vi "Display.vi"(8 "error in":errorcluster, 11 "Input (DBL) in":refnum<class "Input (DBL).lvclass">) -> (0 "error out":errorcluster, 3 "Input (DBL) out":refnum<class "Input (DBL).lvclass">)   [LabVIEW 2021, in "Pop-Up.lvlib" / "Input (DBL).lvclass"]
doc: "This vi will display the input pop up waiting for a type Double input from the user\n\n<b>Code Developed By:</b>\nDaniel Coons\nTechnology Service Corporation\n1983 S Liberty Drive\nBloomington, IN 47403\nPhone: 812 558-7100\ndaniel.coons@tsc.com\nwww.tsc.com/atcs"
uses:
  Input (DBL).lvclass
  C:/Development/Open Source/tsc-pop-up/Popup/Popup.lvclass
  Input (DBL).lvclass/Input (DBL).ctl
  Popup/Popup.lvclass/Popup.ctl
  Popup/Data Member Access/Read Theme.vi
  Theme/Theme.lvclass
  Popup/Popup.lvclass
  user32.dll
panel:
  out "header":bool
  out "2D Picture":picture
  in  "OK Button":bool
  out "Input value out":dbl=1.0 min=1.0 format="%.10g"
  in  "Input":dbl format="%#.10g"
  out "String":string
  # "This VI displays the popup"
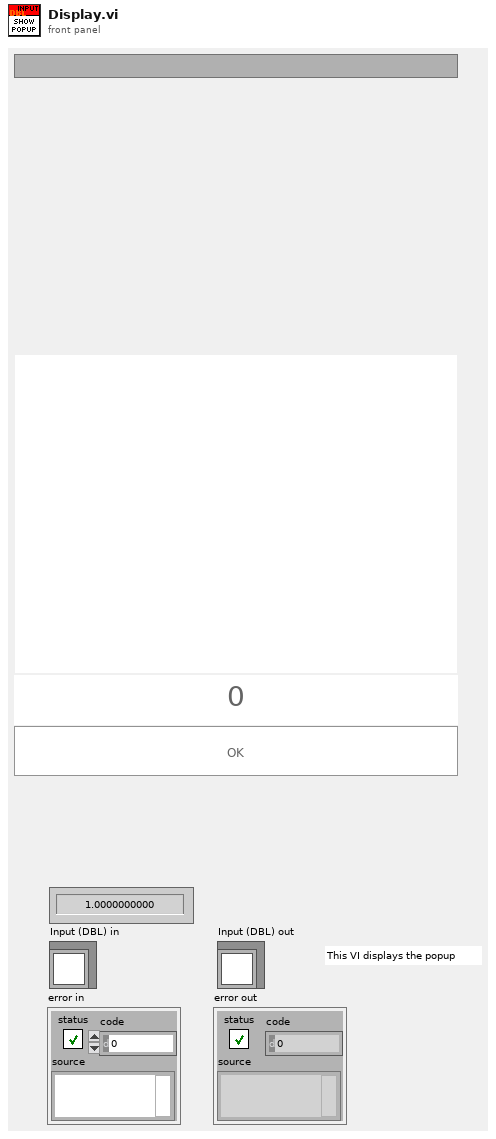
[diagram p1: front panel]
types:
  T1 = typedef "LVPoint32TypeDef.ctl" = cluster{"Horizontal":i32, "Vertical":i32}
  T2 = typedef "LVPositionTypeDef.ctl" = cluster{"Left":i32, "Top":i32}
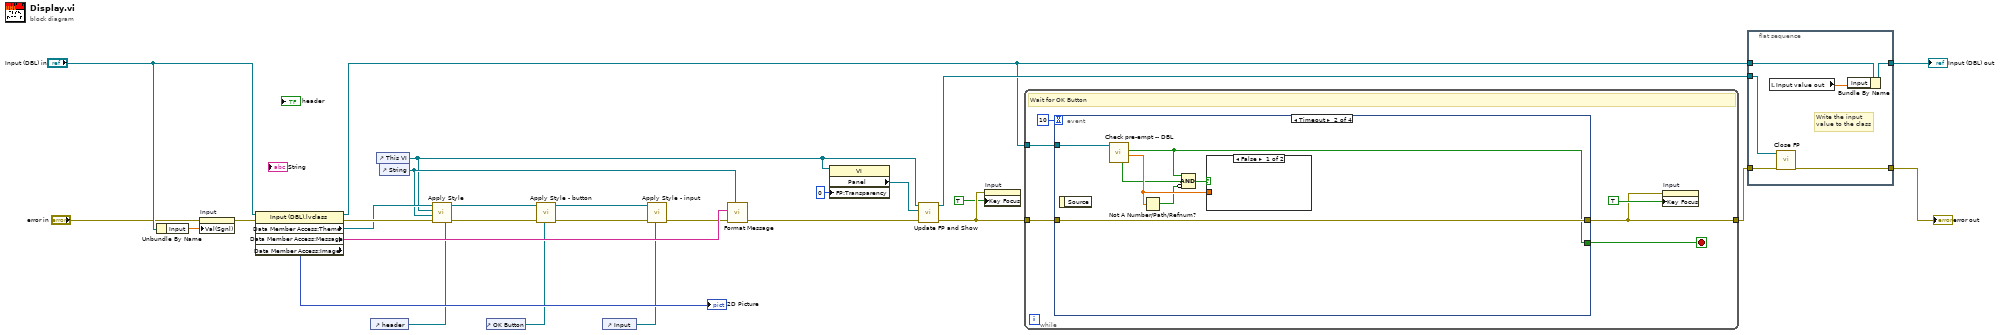
[diagram p0: block diagram]
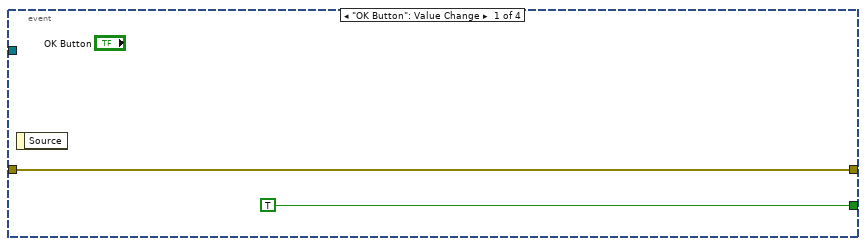
[diagram p2: hidden frame]
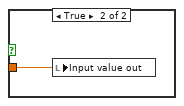
[diagram p3: hidden frame]
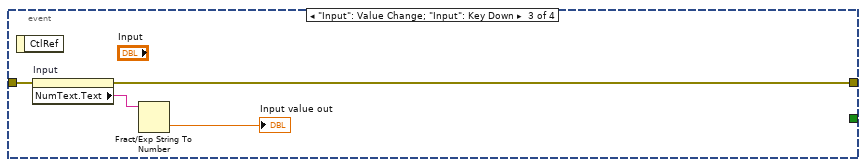
[diagram p4: hidden frame]
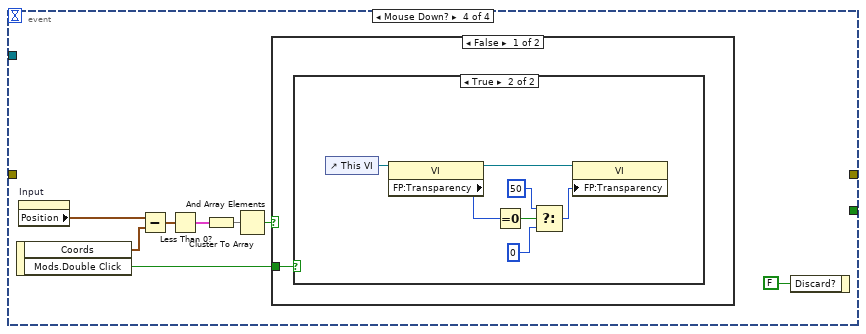
[diagram p5: hidden frame]
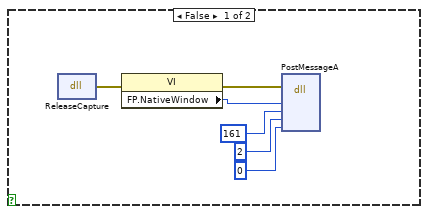
[diagram p6: hidden frame]
diagram:
  n1 = Unbundle By Name("Input (DBL) in") -> ("Input"=w22:dbl)
  n2 = property on="Input" class="DigNum (strict)"(error in="error in", "Val(Sgnl)"=w22) -> (error out=w23:errorcluster)  [unwired: 1 in, 1 out]
  n3 = property class="Input (DBL).lvclass"(reference="Input (DBL) in", error in=w23) -> (reference out=w17:refnum<class "Input (DBL).lvclass">, error out=w14:errorcluster, "Data Member Access:Theme"=w11:refnum<class "Theme.lvclass">, "Data Member Access:Message"=w15:string, "Data Member Access:Image"=→"2D Picture":picture)
  n4 = control-ref of="header"() -> (w8:refnum<vi>)
  n5 = control-ref of="This VI"() -> (w9:refnum<vi>)
  n6 = control-ref of="String"() -> (w10:refnum<vi>)
  n7 = call "Apply Style.vi"("header ref"=w8, "error in"=w14, "message ref"=w10, "pop up ref"=w9, "Theme in"=w11) -> ("error out"=w12:errorcluster, "Theme out"=w6:refnum<class "Theme.lvclass">)  [unwired: 5 in]
  n8 = control-ref of="OK Button"() -> (w5:refnum<vi>)
  n9 = call "Apply Style - button.vi"("button ref"=w5, "error in"=w12, "Theme in"=w6) -> ("error out"=w7:errorcluster, "Theme out"=w3:refnum<class "Theme.lvclass">)  [unwired: 7 in]
  n10 = control-ref of="Input"() -> (w2:refnum<vi>)
  n11 = call "Apply Style - input.vi"("input ref"=w2, "error in (no error)"=w7, "Theme in"=w3) -> ("error out"=w4:errorcluster)  [unwired: 7 in, 1 out]
  n12 = call "Format Message.vi"("formatted string"=w10, "error in"=w4, "String Input"=w15) -> ("error out"=w16:errorcluster)  [unwired: 7 in, 1 out]
  n13 = property class="VI"(reference=w9, "FP:Transparency"=u8 0 ("Front Panel Window:Transparency")) -> ("Panel"=w21:refnum<vi>)  [unwired: 1 in, 2 out]
  n14 = call "Update FP and Show.vi"("error in (no error)"=w16, "Panel Ref"=w21, "VI in"=w9) -> ("error out"=w19:errorcluster, "VI out"=w20:refnum<vi>)  [unwired: 7 in]
  n15 = property on="Input" class="DigNum (strict)"(error in=w19, "Key Focus"=TRUE) -> ()  [unwired: 1 in, 2 out]
  n16 = while {
    tunnel: w19 -> [w34]
    tunnel: [w29] -> w24
    tunnel: w17 -> [w31]
    stop <- w33 stop-if-true
    # "Wait for OK Button"
    n17 = event shown="[1] Timeout" {
      selector: _ -> [_ _ _ _]
      dyn-events: _ -> [_ _ _ _]
      timeout: 10 -> [_ _ _ _]
      tunnel: w34 -> [w36 w43 w48 _]
      tunnel: [w36 w43 w45 _] -> w29
      tunnel: [TRUE w40 _ _] -> w33
      tunnel: w31 -> [_ w42 _ _]
      event "OK Button": Value Change {
        n18 = event-data() -> ()  [unwired: 1 in, 1 out]
      }
      event Timeout {
        n19 = event-data() -> ()  [unwired: 1 in, 1 out]
        n20 = call "Check pre-empt -- DBL.vi"("_Popup in"=w42) -> ("Value?"=w41:dbl, "Pre-empted?"=w40:bool, "Type Match?"=w38:bool)  [unwired: 7 in, 1 out]
        n21 = Not A Number/Path/Refnum?(number/path/refnum=w41) -> (NaN/Path/Refnum?=w37:bool)
        n22 = Compound Arithmetic op=AND(w40, w38, invert w37) -> (w39:bool)
        n23 = case shown="False" w39 {
          tunnel: w41 -> [_ w44]
          frame False {
          }
          frame True {
            n24 = local write "Input value out"(w44) -> ()
          }
        }
      }
      event "Input": Value Change; "Input": Key Down {
        n25 = event-data() -> ()  [unwired: 1 in, 1 out]
        n26 = property on="Input" class="DigNum (strict)"(error in=w48) -> (error out=w45:errorcluster, "NumText.Text"=w47:string)  [unwired: 1 in, 1 out]
        n27 = Fract/Exp String To Number(string=w47) -> (number=→"Input value out":dbl)  [unwired: 3 in, 1 out]
      }
      event Mouse Down? {
        n28 = event-data() -> ("Coords"=w51:T1, "Mods.Double Click"=w49:bool)  [unwired: 1 in]
        n29 = property on="Input" class="DigNum (strict)"() -> ("Position"=w52:T2)  [unwired: 2 in, 2 out]
        n30 = Subtract(x=w52, y=w51) -> (x-y=w53:T2)
        n31 = Less Than 0?(x=w53) -> (x < 0?=w54:cluster{"Left":bool, "Top":bool})
        n32 = Cluster To Array(cluster=w54) -> (array=w55:bool[])
        n33 = And Array Elements(Boolean array=w55) -> (logical AND=w50:bool)
        n34 = case shown="False" w50 {
          tunnel: w49 -> [w57 _]
          frame False {
            n35 = case shown="True" w57 {
              frame False {
                n36 = dll-call lib="user32.dll" fn="ReleaseCapture"() -> (error out=w61:errorcluster)  [unwired: 4 in, 1 out]
                n37 = property class="VI"(error in=w61) -> (error out=w62:errorcluster, "FP.NativeWindow"=w63:u64)  [unwired: 1 in, 1 out]
                n38 = dll-call lib="user32.dll" fn="PostMessageA"(error in=w62, "hWnd"=w63, "Msg"=161, "wParam"=2, "lParam"=0) -> ()  [unwired: 7 in, 2 out]
              }
              frame True {
                n39 = control-ref of="This VI"() -> (w70:refnum<vi>)
                n40 = property class="VI"(reference=w70) -> (reference out=w68:refnum<vi>, "FP:Transparency"=w69:u8)  [unwired: 1 in, 1 out]
                n41 = Equal To 0?(x=w69) -> (x = 0?=w67:bool)
                n42 = Select(t=u8 50, s=w67, f=u8 0) -> (s? t:f=w66:u8)
                n43 = property class="VI"(reference=w68, "FP:Transparency"=w66) -> ()  [unwired: 1 in, 2 out]
              }
            }
          }
          frame True {
          }
        }
        n44 = event-data("Discard?"=FALSE) -> ()  [unwired: 1 in, 1 out]
      }
    }
    n45 = property on="Input" class="DigNum (strict)"(error in=w29, "Key Focus"=TRUE) -> ()  [unwired: 1 in, 2 out]
  }
  n46 = flat-sequence {
    tunnel: w24 -> [w76]
    tunnel: [w72] -> w25
    tunnel: w17 -> [w75]
    tunnel: [w74] -> w26
    tunnel: w20 -> [w71]
    frame #0 {
      # "Write the input\nvalue to the class"
      n47 = local read "Input value out"() -> (w73:dbl)
      n48 = call "Close FP.vi"("error in (no error)"=w76, "VI in"=w71) -> ("error out"=w72:errorcluster)  [unwired: 9 in]
      n49 = Bundle By Name(cluster=w75, "Input"=w73) -> (w74:refnum<class "Input (DBL).lvclass">)
    }
  }
  "error out" <- w25
  "Input (DBL) out" <- w26
